vi "Pack Data and Write to Inline.vi"(8 "Error In":errorcluster, 10 "Injection Event Data Cluster":T1 {"Measurements"."Shots"."Results"."Off-Stage Min Volt" format="%#.6g"; "Measurements"."Shots"."Results"."Off-Stage Avg Volt" format="%#.6g"; "Measurements"."Shots"."Results"."Off-Stage Max Volt" format="%#.6g"; "Measurements"."Shots"."Results"."Total Stage Time (us)" format="%#.6g"; "Measurements"."Shots"."Results"."Off-Stage Avg Current" format="%#.6g"; "Measurements"."Shots"."Results"."Total Voltage Pulses" format="%#.6g"; "Measurements"."Shots"."Results"."Off-Stage Min Current" format="%#.6g"; "Measurements"."Shots"."Results"."Off-Stage Max Current" format="%#.6g"}, 11 "Async Parameters":T4) -> (0 "Error out":errorcluster, 3 "Async Parameters out":T4)   [LabVIEW 2019, in "Fuel Injector Analysis Addon Engine.lvlib"]
uses:
  Fuel Injector Analysis Addon Engine.lvlib
  Types/Async Parameters.ctl
  Addon Shared/Types/Shot.Parameters.ctl
  Addon Shared/Types/Stage.Parameters.ctl
  Addon Shared/Types/Stage.PullIn.Types.ctl
  Addon Shared/Types/Stage.Transition.Types.ctl
  Addon Shared/Types/Analysis.Channels.Select.ctl
  Addon Shared/Types/Injector info.ctl
  Types/Injector.State.ctl
  <vilib>/NI/NIVS Inline Async API/_Data Access Engine/Data Access Engine/Types/Write.DVR.ctl
  <vilib>/NI/NIVS Inline Async API/_Data Access Engine/Access Type Classes/Write/Write.lvclass
  <vilib>/NI/NIVS Inline Async API/_Data Access Engine/Data Access Engine/Types/Read.DVR.ctl
  <vilib>/NI/NIVS Inline Async API/_Data Access Engine/Access Type Classes/Read/Read.lvclass
  Addon Shared/Types/Compiled.Group.WaveformRefs.ctl
  <vilib>/NI VeriStand/Custom Device API/Waveform Data Reference.ctl
  <vilib>/NI VeriStand/Custom Device Waveform API/Single Waveform Write (DBL)/Single Waveform Write (DBL).lvclass
  Types/Injector Event Data Cluster.ctl
  Types/Shot Information Control.ctl
  Types/Stage.Measurements.ctl
  <vilib>/NI/NIVS Inline Async API/_Data Access Engine/Access Type Classes/Write/Write.lvclass/Write.ctl
  <vilib>/NI/NIVS Inline Async API/_Data Access Engine/Data Access Engine/Methods/Write.Data.vi
  <vilib>/NI/NIVS Inline Async API/_Data Access Engine/Access Type Classes/Write/Write.ProcessData.vi
  <vilib>/NI/NIVS Inline Async API/_Data Access Engine/Access Type Classes/Write/Write.Buffer.vi
  <vilib>/NI/NIVS Inline Async API/_Data Access Engine/Access Type Classes/Write/Write.Commit.vi
  <vilib>/NI/NIVS Inline Async API/_Data Access Engine/Data Access Engine/Data Access Engine.lvclass
  Addon Shared/Fuel Injector Analysis Addon Shared.lvlib
  <vilib>/NI VeriStand/Custom Device API/Custom Device API.lvlib
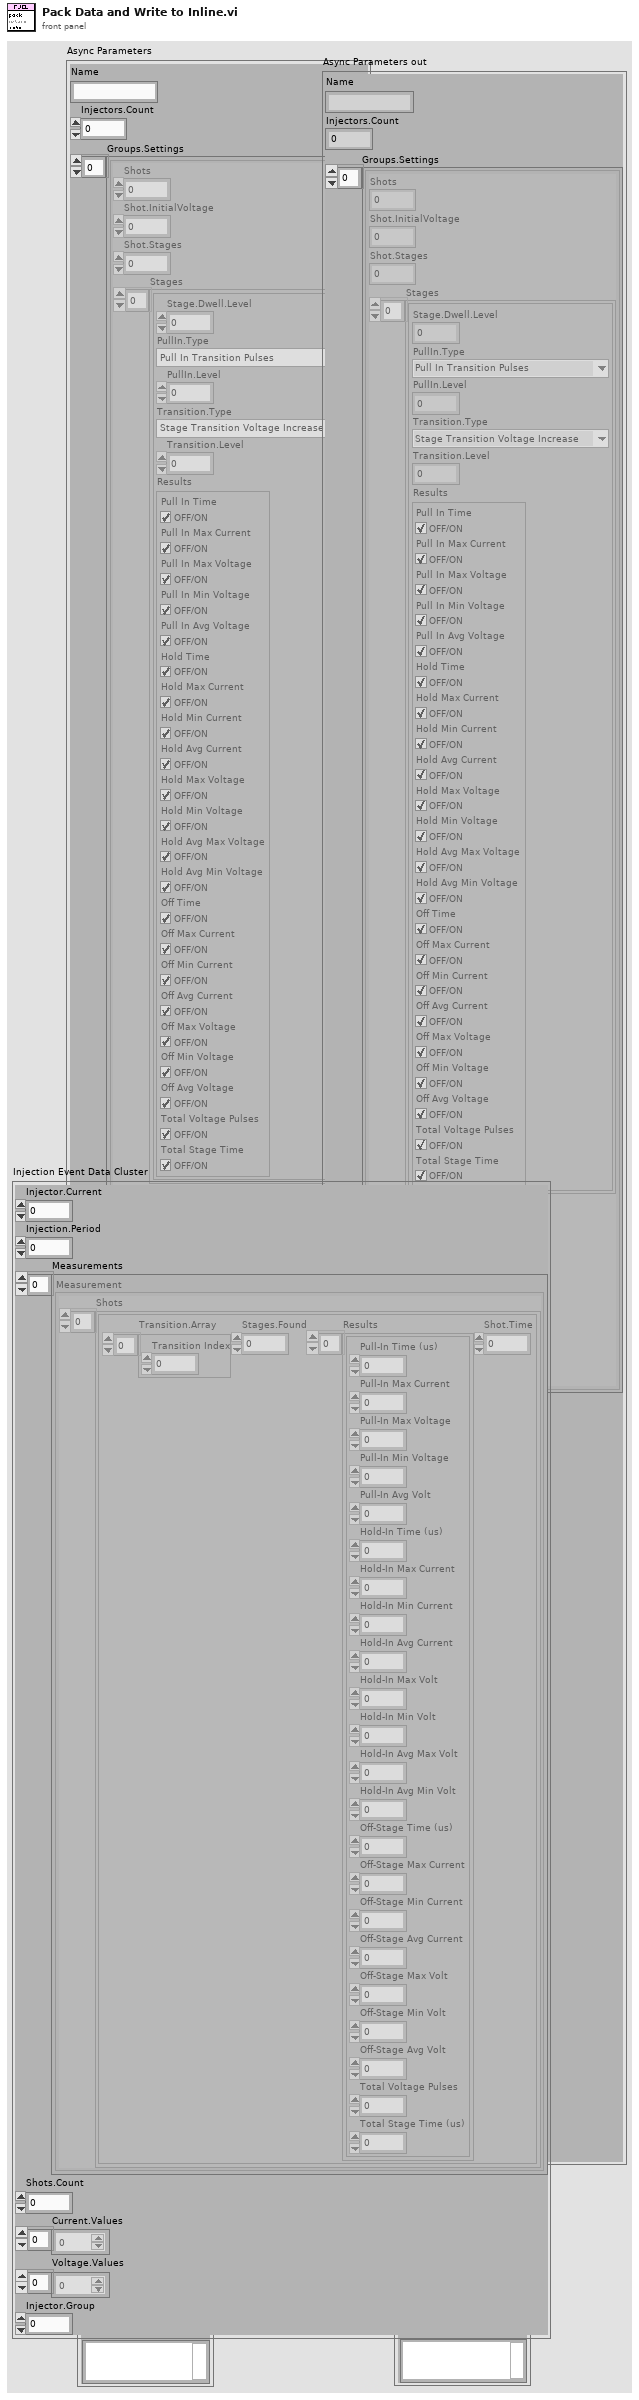
[diagram p1: front panel]
types:
  T1 = typedef "Fuel Injector Analysis Addon Engine.lvlib/Injector Event Data Cluster.ctl" = cluster{"Injector.Current":i16, "Injection.Period":dbl, "Measurements":cluster{"Shots":T2[]}[], "Shots.Count":i32, "Current.Values":dbl[], "Voltage.Values":dbl[], "Injector.Group":i16}
  T2 = typedef "Fuel Injector Analysis Addon Engine.lvlib/Shot Information Control.ctl" = cluster{"Transition.Array":i32[], "Stages.Found":u16, "Results":T3[], "Shot.Time":dbl}
  T3 = typedef "Fuel Injector Analysis Addon Engine.lvlib/Stage.Measurements.ctl" = cluster{"Pull-In Time (us)":dbl, "Pull-In Max Current":dbl, "Pull-In Max Voltage":dbl, "Pull-In Min Voltage":dbl, "Pull-In Avg Volt":dbl, "Hold-In Time (us)":dbl, "Hold-In Max Current":dbl, "Hold-In Min Current":dbl, "Hold-In Avg Current":dbl, "Hold-In Max Volt":dbl, "Hold-In Min Volt":dbl, "Hold-In Avg Max Volt":dbl, "Hold-In Avg Min Volt":dbl, "Off-Stage Time (us)":dbl, "Off-Stage Max Current":dbl, "Off-Stage Min Current":dbl, "Off-Stage Avg Current":dbl, "Off-Stage Max Volt":dbl, "Off-Stage Min Volt":dbl, "Off-Stage Avg Volt":dbl, "Total Voltage Pulses":dbl, "Total Stage Time (us)":dbl}
  T4 = typedef "Fuel Injector Analysis Addon Engine.lvlib/Async Parameters.ctl" = cluster{"Name":string, "Injectors.Count":u8, "Groups.Settings":T5[], "Groups.InitResults":cluster{"Values":dbl[]}[], "Injectors.Settings":T10[], "Injectors.State":T11[], "DMA.Ref":refnum<k20>, "FPGA.Status":T12, "Search.Data":T13, "Results.Data":T12, "Waveform.Enable":T13, "Waveform.Refs":T14[], "Waveform.Sessions":refnum<class "Single Waveform Write (DBL).lvclass">[]}
  T5 = typedef "Fuel Injector Analysis Addon Shared.lvlib/Shot.Parameters.ctl" = cluster{"Shots":u32, "Shot.InitialVoltage":dbl, "Shot.Stages":u32, "Stages":T6[], "Timeout":dbl, "Results.Count":i32, "Active Edge":bool, "Rate.Hz":u32, "Channels":u32}
  T6 = typedef "Fuel Injector Analysis Addon Shared.lvlib/Stage.Parameters.ctl" = cluster{"Stage.Dwell.Level":dbl, "PullIn.Type":T7, "PullIn.Level":dbl, "Transition.Type":T8, "Transition.Level":dbl, "Results":T9}
  T7 = typedef "Fuel Injector Analysis Addon Shared.lvlib/Stage.PullIn.Types.ctl" = enum8{"Pull In Transition Pulses", "Pull In Transition Current Drop"}
  T8 = typedef "Fuel Injector Analysis Addon Shared.lvlib/Stage.Transition.Types.ctl" = enum8{"Stage Transition Inactive Time", "Stage Transition Voltage Increase", "Stage Transition Current Decrease", "Stage Transition Active Time"}
  T9 = typedef "Fuel Injector Analysis Addon Shared.lvlib/Analysis.Channels.Select.ctl" = cluster{"Pull In Time":bool, "Pull In Max Current":bool, "Pull In Max Voltage":bool, "Pull In Min Voltage":bool, "Pull In Avg Voltage":bool, "Hold Time":bool, "Hold Max Current":bool, "Hold Min Current":bool, "Hold Avg Current":bool, "Hold Max Voltage":bool, "Hold Min Voltage":bool, "Hold Avg Max Voltage":bool, "Hold Avg Min Voltage":bool, "Off Time":bool, "Off Max Current":bool, "Off Min Current":bool, "Off Avg Current":bool, "Off Max Voltage":bool, "Off Min Voltage":bool, "Off Avg Voltage":bool, "Total Voltage Pulses":bool, "Total Stage Time":bool}
  T10 = typedef "Fuel Injector Analysis Addon Shared.lvlib/Injector info.ctl" = cluster{"Results Index":i32, "Waveform Index":i32, "Group":u16}
  T11 = typedef "Fuel Injector Analysis Addon Engine.lvlib/Injector.State.ctl" = cluster{"Timer":u32, "Events":u64}
  T12 = typedef "Data Access Engine.lvlib/Data Access Engine.lvclass/Write.DVR.ctl" = refnum<data-value>
  T13 = typedef "Data Access Engine.lvlib/Data Access Engine.lvclass/Read.DVR.ctl" = refnum<data-value>
  T14 = typedef "Fuel Injector Analysis Addon Shared.lvlib/Compiled.Group.WaveformRefs.ctl" = cluster{"WaveformRefs":T15[], "Group":i32}
  T15 = typedef "Custom Device API.lvlib/Waveform Data Reference.ctl" = i32
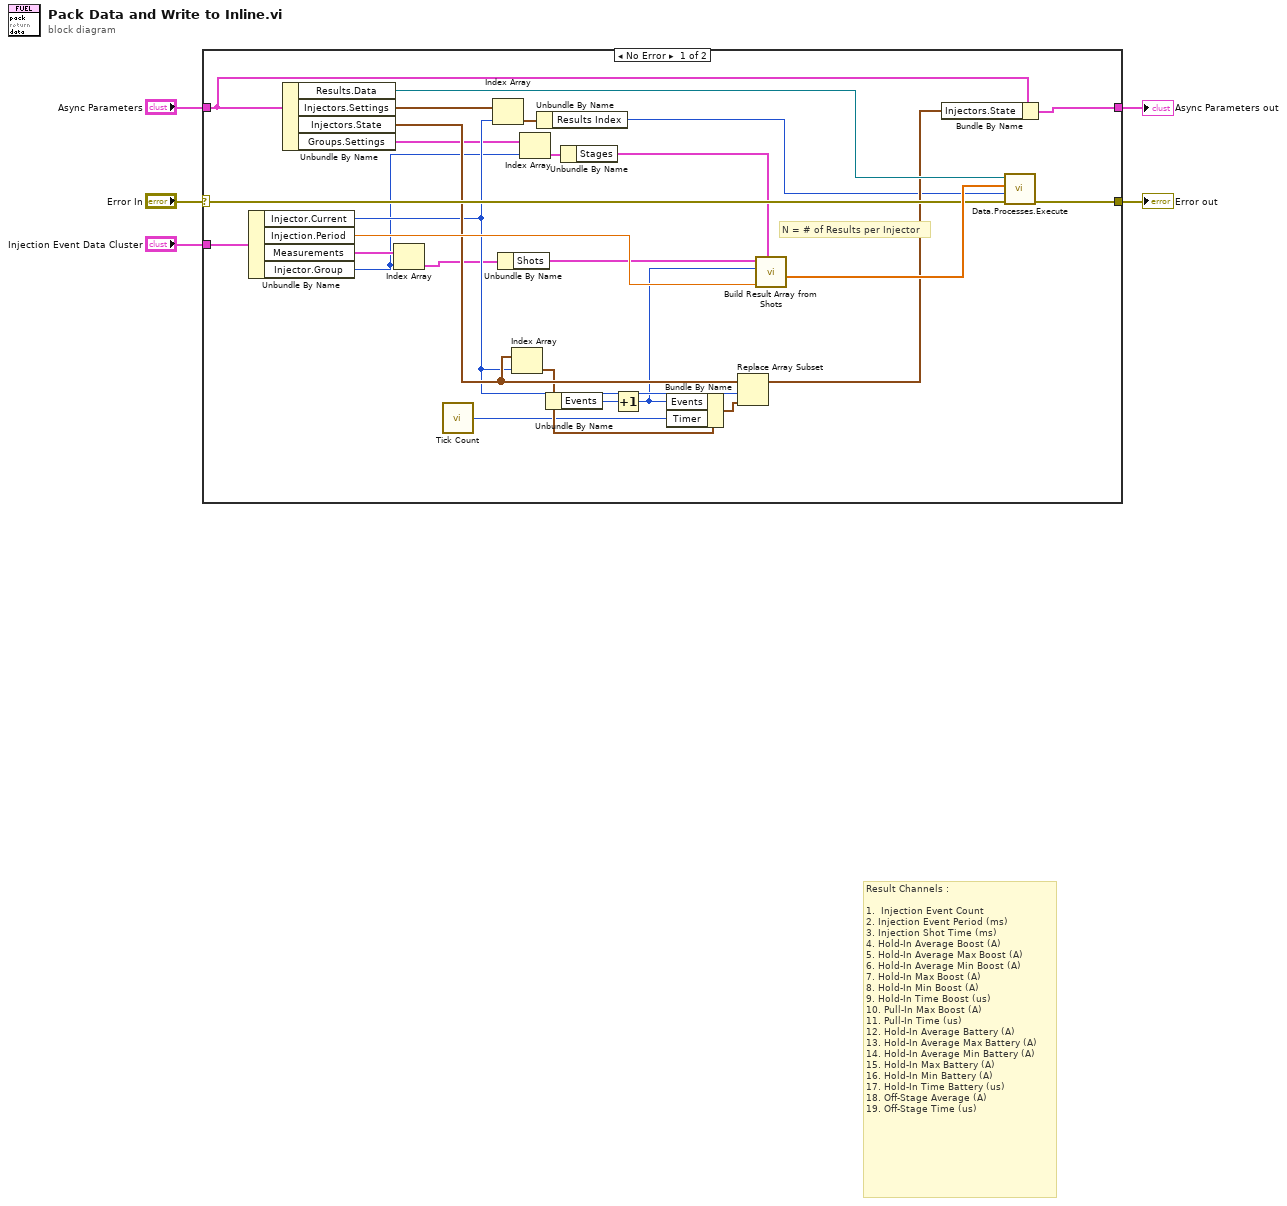
[diagram p0: block diagram]
diagram:
  # "Result Channels :\n\n1.  Injection Event Count\n2. Injection Event Period (ms)\n3. Injection Shot Time (ms)\n4. Hold-In Average Boost (A)\n5. Hold-In Average Max Boost (A)\n6. Hold-In Average Min Boost (A)\n7. Hold-In Max Boost (A)\n8. Hold-In Min Boost (A)\n9. Hold-In Time Boost (us)\n10. Pull-In Max Boost (A)\n11. Pull-In Time (us)\n12. Hold-In Average Battery (A)\n13. Hold-In Average Max Battery (A)\n14. Hold-In Average Min Battery (A)\n15. Hold-In Max Battery (A)\n16. Hold-In Min Battery (A)\n17. Hold-In Time Battery (us)\n18. Off-Stage Average (A)\n19. Off-Stage Time (us)"
  n1 = case shown="No Error" "Error In" {
    selector: "Error In" -> [w26 w33]
    tunnel: [w31 w33] -> w3
    tunnel: "Async Parameters" -> [w24 w32]
    tunnel: [w23 w32] -> w2
    tunnel: "Injection Event Data Cluster" -> [w29 _]
    frame No Error {
      # "N = # of Results per Injector"
      n2 = Unbundle By Name(w29) -> ("Injector.Current"=w18:i16, "Injection.Period"=w28:dbl, "Measurements"=w17:cluster{"Shots":T2[]}[], "Injector.Group"=w14:i16)
      n3 = Unbundle By Name(w24) -> ("Results.Data"=w30:T12, "Injectors.Settings"=w21:T10[], "Injectors.State"=w25:T11[], "Groups.Settings"=w12:T5[])
      n4 = Index Array(array=w17, index=w14) -> (element=w16:cluster{"Shots":T2[]})
      n5 = call "Tick Count"() -> ("Tick Count(mSec)"=w6:u32)
      n6 = Index Array(array=w21, index=w18) -> (element=w20:T10)
      n7 = Unbundle By Name(w16) -> ("Shots"=w15:T2[])
      n8 = Index Array(array=w25, index=w18) -> (element=w9:T11)
      n9 = Index Array(array=w12, index=w14) -> (element=w13:T5)
      n10 = Unbundle By Name(w20) -> ("Results Index"=w19:i32)
      n11 = Unbundle By Name(w9) -> ("Events"=w10:u64)
      n12 = Unbundle By Name(w13) -> ("Stages"=w11:T6[])
      n13 = Increment(x=w10) -> (x+1=w8:u64)
      n14 = Bundle By Name(cluster=w9, "Events"=w8, "Timer"=w6) -> (w7:T11)
      n15 = Replace Array Subset(array=w25, new element=w7, index=w18) -> (w22:T11[])
      n16 = call "Build Result Array from Shots.vi"("Stages"=w11, "Injection Event Dwell Period (ms)"=w28, "Injection Event Count"=w8, "Shot Info Array"=w15) -> ("Result Array"=w27:dbl[])  [unwired: 7 in]
      n17 = Bundle By Name(cluster=w24, "Injectors.State"=w22) -> (w23:T4)
      n18 = call-poly <vilib>:"Data.Processes.Execute.vi"("error in (no error)"=w26, "Offset"=w19, "Values"=w27, "Ref"=w30) -> ("error out"=w31:errorcluster)  [unwired: 7 in]
    }
    frame Error {
    }
  }
  "Error out" <- w3
  "Async Parameters out" <- w2
